vi "get_frequencies.vi"(8 "error in (no error)":errorcluster, 11 "TrajectoryTS090820Circular2D in":refnum<class "TrajectoryTS090820Circular2D.lvclass">) -> (0 "error out":errorcluster, 1 "y frequency":dbl, 2 "x frequency":dbl, 3 "TrajectoryTS090820Circular2D out":refnum<class "TrajectoryTS090820Circular2D.lvclass">)   [LabVIEW 2010, in "TrajectoryTS090820Circular2D.lvclass"]
uses:
  TrajectoryTS090820Circular2D.lvclass
  TrajectoryTS090820Circular2D.lvclass/TrajectoryTS090820Circular2D.ctl
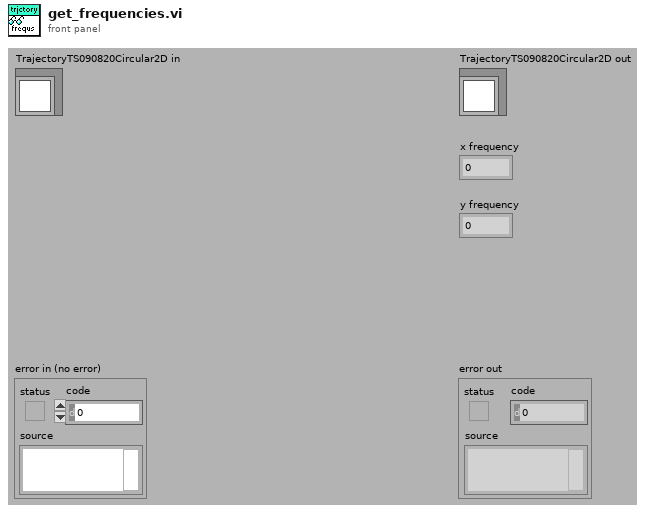
[diagram p1: front panel]
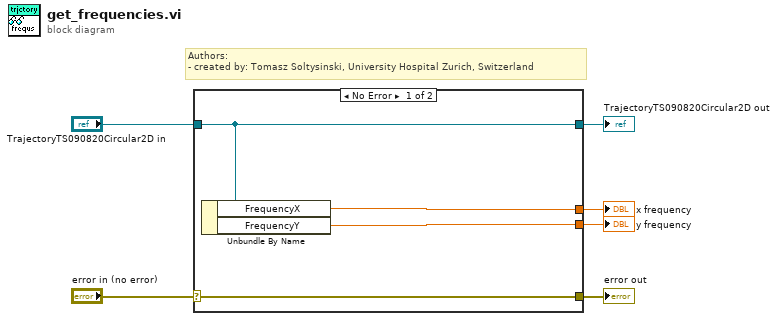
[diagram p0: block diagram]
diagram:
  # "Authors: \n- created by: Tomasz Soltysinski, University Hospital Zurich, Switzerland"
  n1 = case shown="No Error" "error in (no error)" {
    selector: "error in (no error)" -> [w10 w11]
    tunnel: [w10 w11] -> w5
    tunnel: [w9 w12] -> w3
    tunnel: "TrajectoryTS090820Circular2D in" -> [w9 w12]
    tunnel: [w8 _] -> w2
    tunnel: [w7 _] -> w1
    frame No Error {
      n2 = Unbundle By Name(w9) -> ("FrequencyX"=w8:dbl, "FrequencyY"=w7:dbl)
    }
    frame Error {
    }
  }
  "error out" <- w5
  "TrajectoryTS090820Circular2D out" <- w3
  "x frequency" <- w2
  "y frequency" <- w1
